vi "niFpga wdp fft 4-wire wrapper 4spc.vi"(0 "real data in":fxp<+/-,8,1>[](array[numeric])=[0.0, 0.0, 0.0, 0.0], 1 "reset":bool, 5 "imaginary data in":fxp<+/-,8,1>[](array[numeric])=[0.0, 0.0, 0.0, 0.0], 9 "input valid":bool, 12 "ready for output":bool) -> (3 "data indices":u16[](array[numeric]), 4 "real data out":fxp<+/-,19,12>[](array[numeric]), 6 "imaginary data out":fxp<+/-,19,12>[](array[numeric]), 10 "output valid":bool, 14 "ready for input":bool)   [LabVIEW 2017]
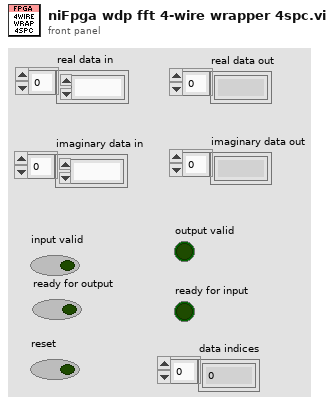
[diagram p1: front panel]
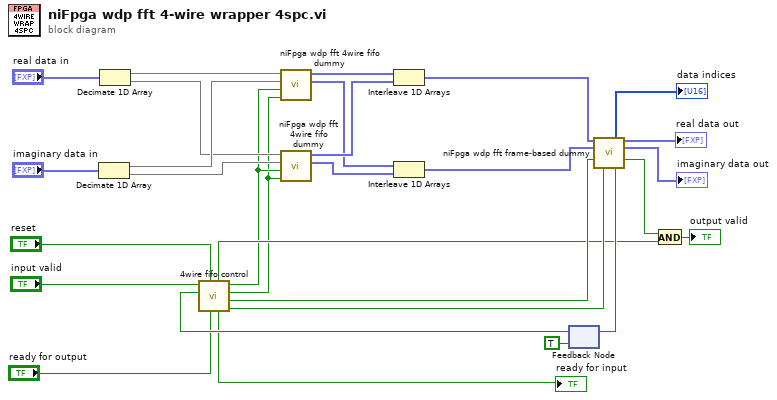
[diagram p0: block diagram]
diagram:
  n1 = Decimate 1D Array("imaginary data in") -> (w19:fxp<+/-,8,1>[], w17:fxp<+/-,8,1>[])
  n2 = Decimate 1D Array("real data in") -> (w20:fxp<+/-,8,1>[], w18:fxp<+/-,8,1>[])
  n3 = feedback #1(TRUE ("ready for frame")) -> (w8:bool)
  n4 = call "4wire fifo control"("ready for output"="ready for output", "reset"="reset", "ready for frame"=w8, "input valid"="input valid") -> ("enable"=w10:bool, "frame start"=w9:bool, "read?"=w1:bool, "write?"=w2:bool, "ready for input"=→"ready for input":bool, "not in reset?"=w3:bool)  [unwired: 2 in]
  n5 = call <vilib>:"niFpga wdp fft 4wire fifo dummy.vi"("read?"=w1, "write?"=w2, "data in im"=w19, "data in re"=w20) -> ("data out im"=w13:fxp<+/-,8,1>[], "data out re"=w16:fxp<+/-,8,1>[])  [unwired: 6 in]
  n6 = call <vilib>:"niFpga wdp fft 4wire fifo dummy.vi"("read?"=w1, "write?"=w2, "data in im"=w17, "data in re"=w18) -> ("data out im"=w12:fxp<+/-,8,1>[], "data out re"=w15:fxp<+/-,8,1>[])  [unwired: 6 in]
  n7 = Interleave 1D Arrays(w16, w15) -> (w14:fxp<+/-,8,1>[])
  n8 = Interleave 1D Arrays(w13, w12) -> (w11:fxp<+/-,8,1>[])
  n9 = call <vilib>:"niFpga wdp fft frame-based dummy.vi"("real data in"=w14, "imaginary data in"=w11, "input frame start"=w9, "enable"=w10) -> ("data indices"=→"data indices":u16[], "real data out"=→"real data out":fxp<+/-,19,12>[], "imaginary data out"=→"imaginary data out":fxp<+/-,19,12>[], "output valid"=w24:bool, "ready for frame"=w25:bool)  [unwired: 6 in, 1 out]
  n10 = feedback-in #1(w25) -> ()
  n11 = And(x=w24, y=w3) -> (x .and. y?=→"output valid":bool)
